vi "Self-Test.vi"(8 "error in (no error)":errorcluster, 11 "PXIe5105 in":refnum<class "PXIe5105.lvclass">) -> (0 "error out":errorcluster, 2 "Self-Test Passed? (T:Yes)":bool, 3 "PXIe5105 out":refnum<class "PXIe5105.lvclass">)   [LabVIEW 2018, in "PXIe5105.lvlib" / "PXIe5105.lvclass"]
doc: "This Override method is used to call the Self-Test function of the Oscope instrument. The boolean output 'Self-Test Passed? (T:Yes)' carries out the Self-Test result."
uses:
  PXIe5105.lvclass
  PXIe5105.lvclass/PXIe5105.ctl
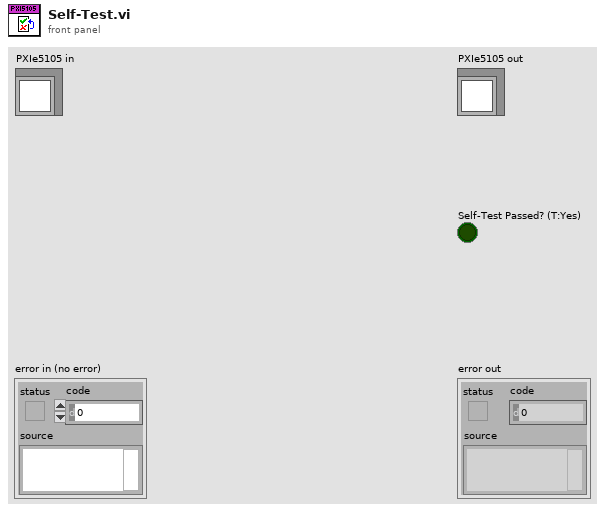
[diagram p1: front panel]
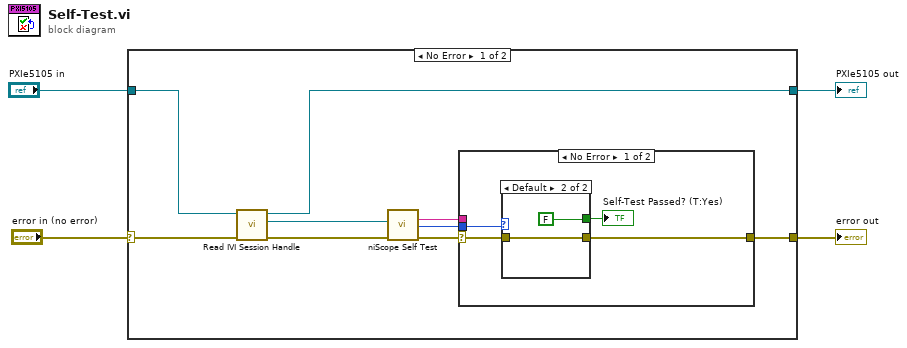
[diagram p0: block diagram]
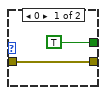
[diagram p2: hidden frame]
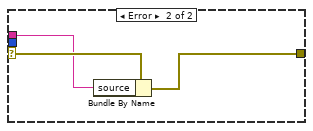
[diagram p3: hidden frame]
diagram:
  n1 = case shown="No Error" "error in (no error)" {
    selector: "error in (no error)" -> [w7 w26]
    tunnel: [w11 w26] -> w3
    tunnel: "PXIe5105 in" -> [w9 w25]
    tunnel: [w8 w25] -> w1
    frame No Error {
      n2 = call "Read IVI Session Handle.vi"("error in (no error)"=w7, "PXIe5105 in"=w9) -> ("error out"=w6:errorcluster, "IVI Session Handle"=w5:refnum<k15>, "PXIe5105 out"=w8:refnum<class "PXIe5105.lvclass">)  [unwired: 7 in]
      n3 = call <instrlib>:"niScope Self Test.vi"("instrument handle"=w5, "error in"=w6) -> ("self-test message"=w12:string, "self test result"=w10:i16, "error out"=w13:errorcluster)  [unwired: 10 in, 1 out]
      n4 = case shown="No Error" w13 {
        selector: w13 -> [w16 w24]
        tunnel: [w15 w22] -> w11
        tunnel: w12 -> [_ w23]
        tunnel: w10 -> [w17 _]
        frame No Error {
          n5 = case shown="Default" w17 {
            tunnel: w16 -> [w19 w20]
            tunnel: [w19 w20] -> w15
            tunnel: [TRUE FALSE] -> w14
            frame 0 {
            }
            frame Default {
            }
          }
          "Self-Test Passed? (T:Yes)" <- w14
        }
        frame Error {
          n6 = Bundle By Name(cluster=w24, "source"=w23) -> (w22:errorcluster)
        }
      }
    }
    frame Error {
    }
  }
  "error out" <- w3
  "PXIe5105 out" <- w1
